vi "main.vi"() -> ()   [LabVIEW 2023]
uses:
  <vilib>/express/express signal manip/GetorSetDDTAttributes/Shared VIs/TimeType.ctl
  5948bca3-3d14-40bf-9fbb-2ba5c3eee3bd.vi
  <vilib>/Analysis/baseanly.llb/Mean (DBL).vi
  faa81322-6883-41b3-8229-1eb533283c0b.vi
  <extravilib>/ChannelInstances/Tag-bool/Read With Abort.vi
  <extravilib>/ChannelInstances/Tag-bool/Write With Abort.vi
  <extravilib>/ChannelInstances/Tag-bool/Instantiate.vi
  <extravilib>/ChannelInstances/Tag-bool/EndpointRead.vi
  <vilib>/express/express signal manip/GetorSetDDTAttributes/Shared VIs/TimeMode Enum to Boolean.vi
  <vilib>/express/express shared/transition.llb/Dynamic To Waveform Array.vi
  <vilib>/express/express signal manip/GetorSetDDTAttributes/Set DDT Attributes/SetT0.vi
  <vilib>/express/express shared/transition.llb/Waveform Array To Dynamic.vi
  <extravilib>/ChannelInstances/Tag-bool/Endpoint.vi
  <vilib>/express/express signal manip/GetorSetDDTAttributes/Set DDT Attributes/Set DDT Properties.xnode
  <extravilib>/ChannelInstances/Tag-bool.lvlib
  <vilib>/ptbypt/NI_PtbyPt.lvlib
  <vilib>/Analysis/NI_AALBase.lvlib
  <vilib>/express/express signal manip/GetorSetDDTAttributes/Shared VIs/GetSetShared.lvlib
panel:
  out "dt":dbl
  in  "?":T1(tab)
  in  "Test Knob":dbl(knob) scale=0.0..10.0
  out "Signal Frequency\n 2":dbl(graph)
  out "Stable RPM measurement?":bool
  in  "Nominal R":dbl
  in  "Nominal Omega":dbl
  in  "Sample rate":dbl=1000.0
  in  "Number of Samples":dbl=5.0
  in  "Voltage Threshold":dbl=0.5
  in  "Number of magnets":dbl=1.0
  out "Omega [RPM]":dbl(knob) scale=0.0..2000.0
  out "Voltage RMS [V]":dbl(knob) scale=0.0..20.0
  out "Power Output [W]":dbl(knob) scale=0.0..20.0
  out "Current RMS [A]":dbl(knob) scale=0.0..20.0
  in  "Button":bool
  out "Signal\nFrequency (Hz)":dbl
  in  "?":bool
  in  "Button 2":bool
  out "Python Error Status":errorcluster
  in  "Filename":path=path "C:/Users/johan/OneDrive - Estudiantes ITCR/TEC/ProyectodeGraduacion/LabEolicaControl/rawdata.txt"
  out "Voltage Sensor":dynamicdata(graph)
  out "Current Sensor":dynamicdata(graph)
  out "Hall sensor\n 2":dynamicdata(graph)
  out "Hall sensor":dynamicdata(graph)
  # "Lab Setup"
  # "Post Processing"
  # "Data Monitoring"
  # "Real Time Analysis variables"
  # "Measurement Point"
  # "File I/O"
  # "About:"
  # "Software Requirements:"
  # "This measuring system was designed for data acquisition of \npower, angular speed, and resistance data for small scale HAWT \nand possibly VAWT. These turbines are being researched and \ndeveloped at LIENE (Laboratorio de Investigación en Energía Eólica) \nat ITCR. \n\nThis module runs a simulation of the measurement signals to test code previous to usage"
  # "Python 3.6+  with the following packages:\n-- NumPy\n-- Plotly"
  # "Programmer:"
  # "This software was designed and programmed by: \n-- Johansell Villalobos Cubillo: \n         Engineering Physics student\n&\n--Mauricio Bolivar Gonzalez"
  # "DAQ Equipment: NI-USB-6000"
  # "The equipment pinout diagram is shown below and the pins are used as follows: \n\nAl 0 -- Hall effect sensor\nAl 1 -- Voltage from zenner diode\nAl 2 -- ACS712 20A current sensor\nAl GND -- common ground"
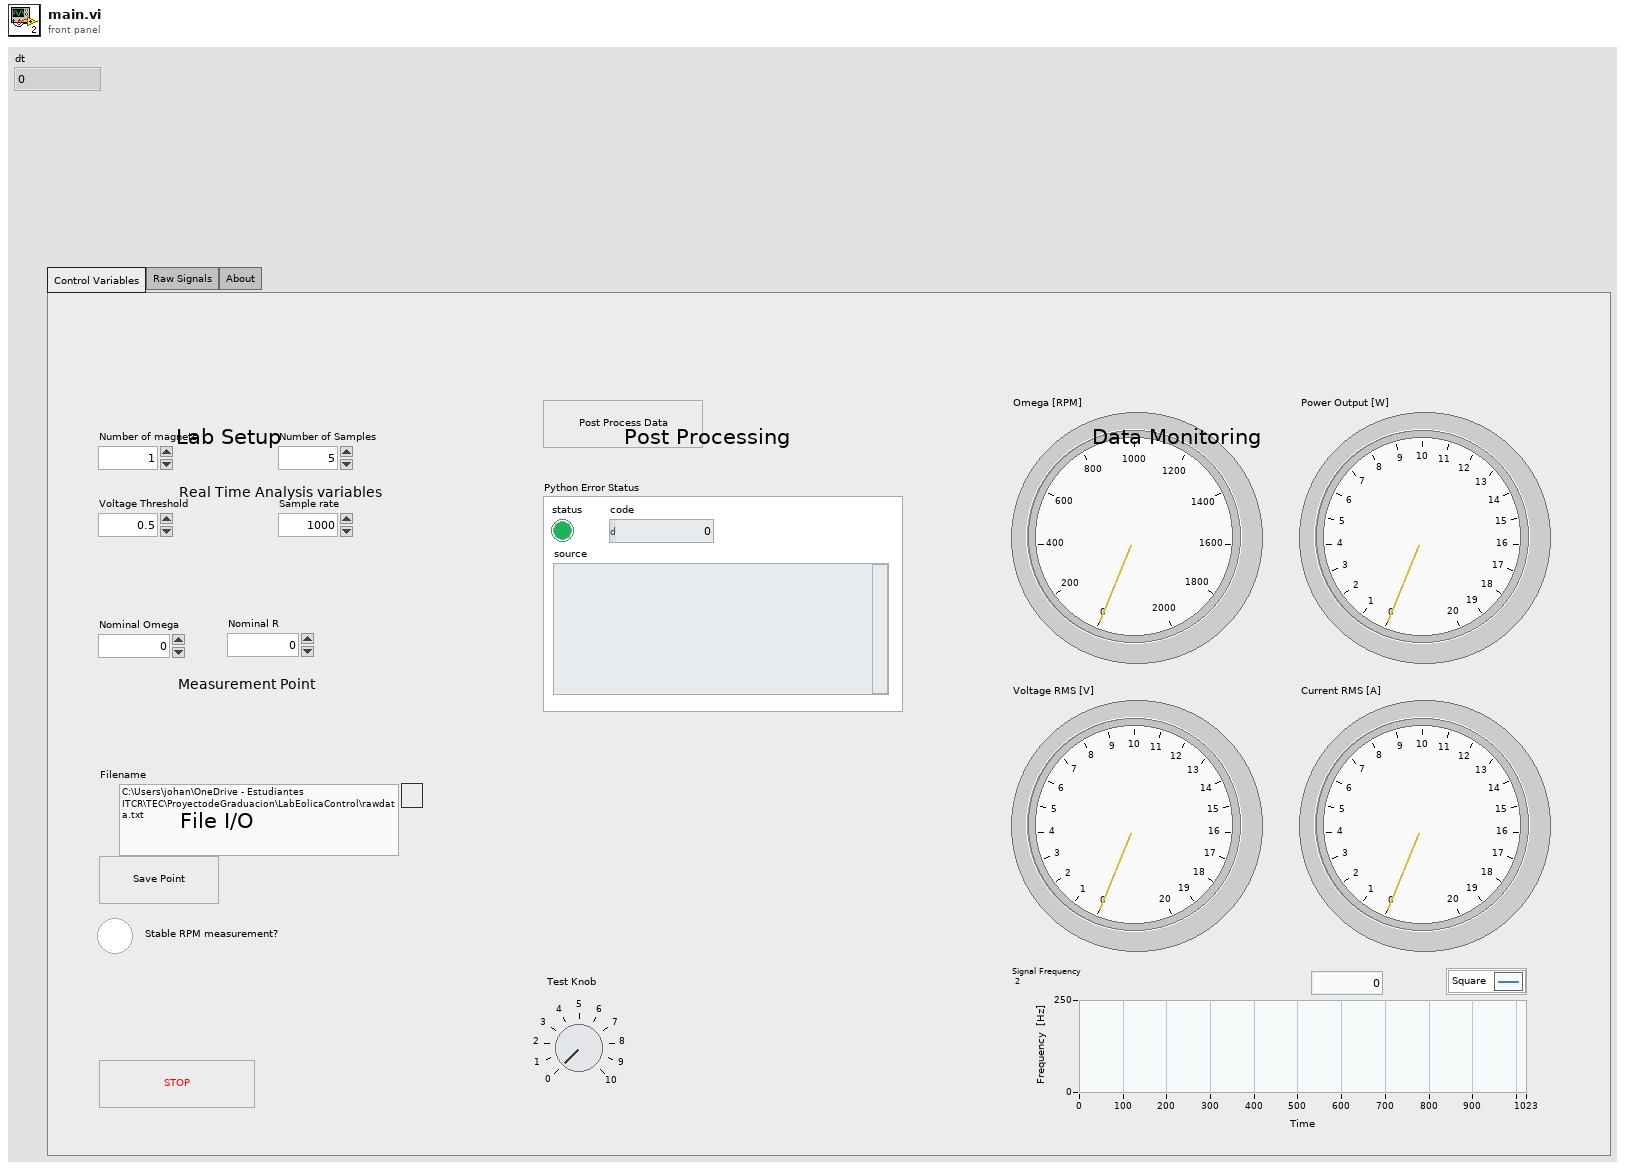
[diagram p1: front panel]
types:
  T1 = enum32{"Control Variables", "Raw Signals", "About"}
  T2 = typedef "Tag-bool.lvlib/))Channel.ctl" = refnum<queue>
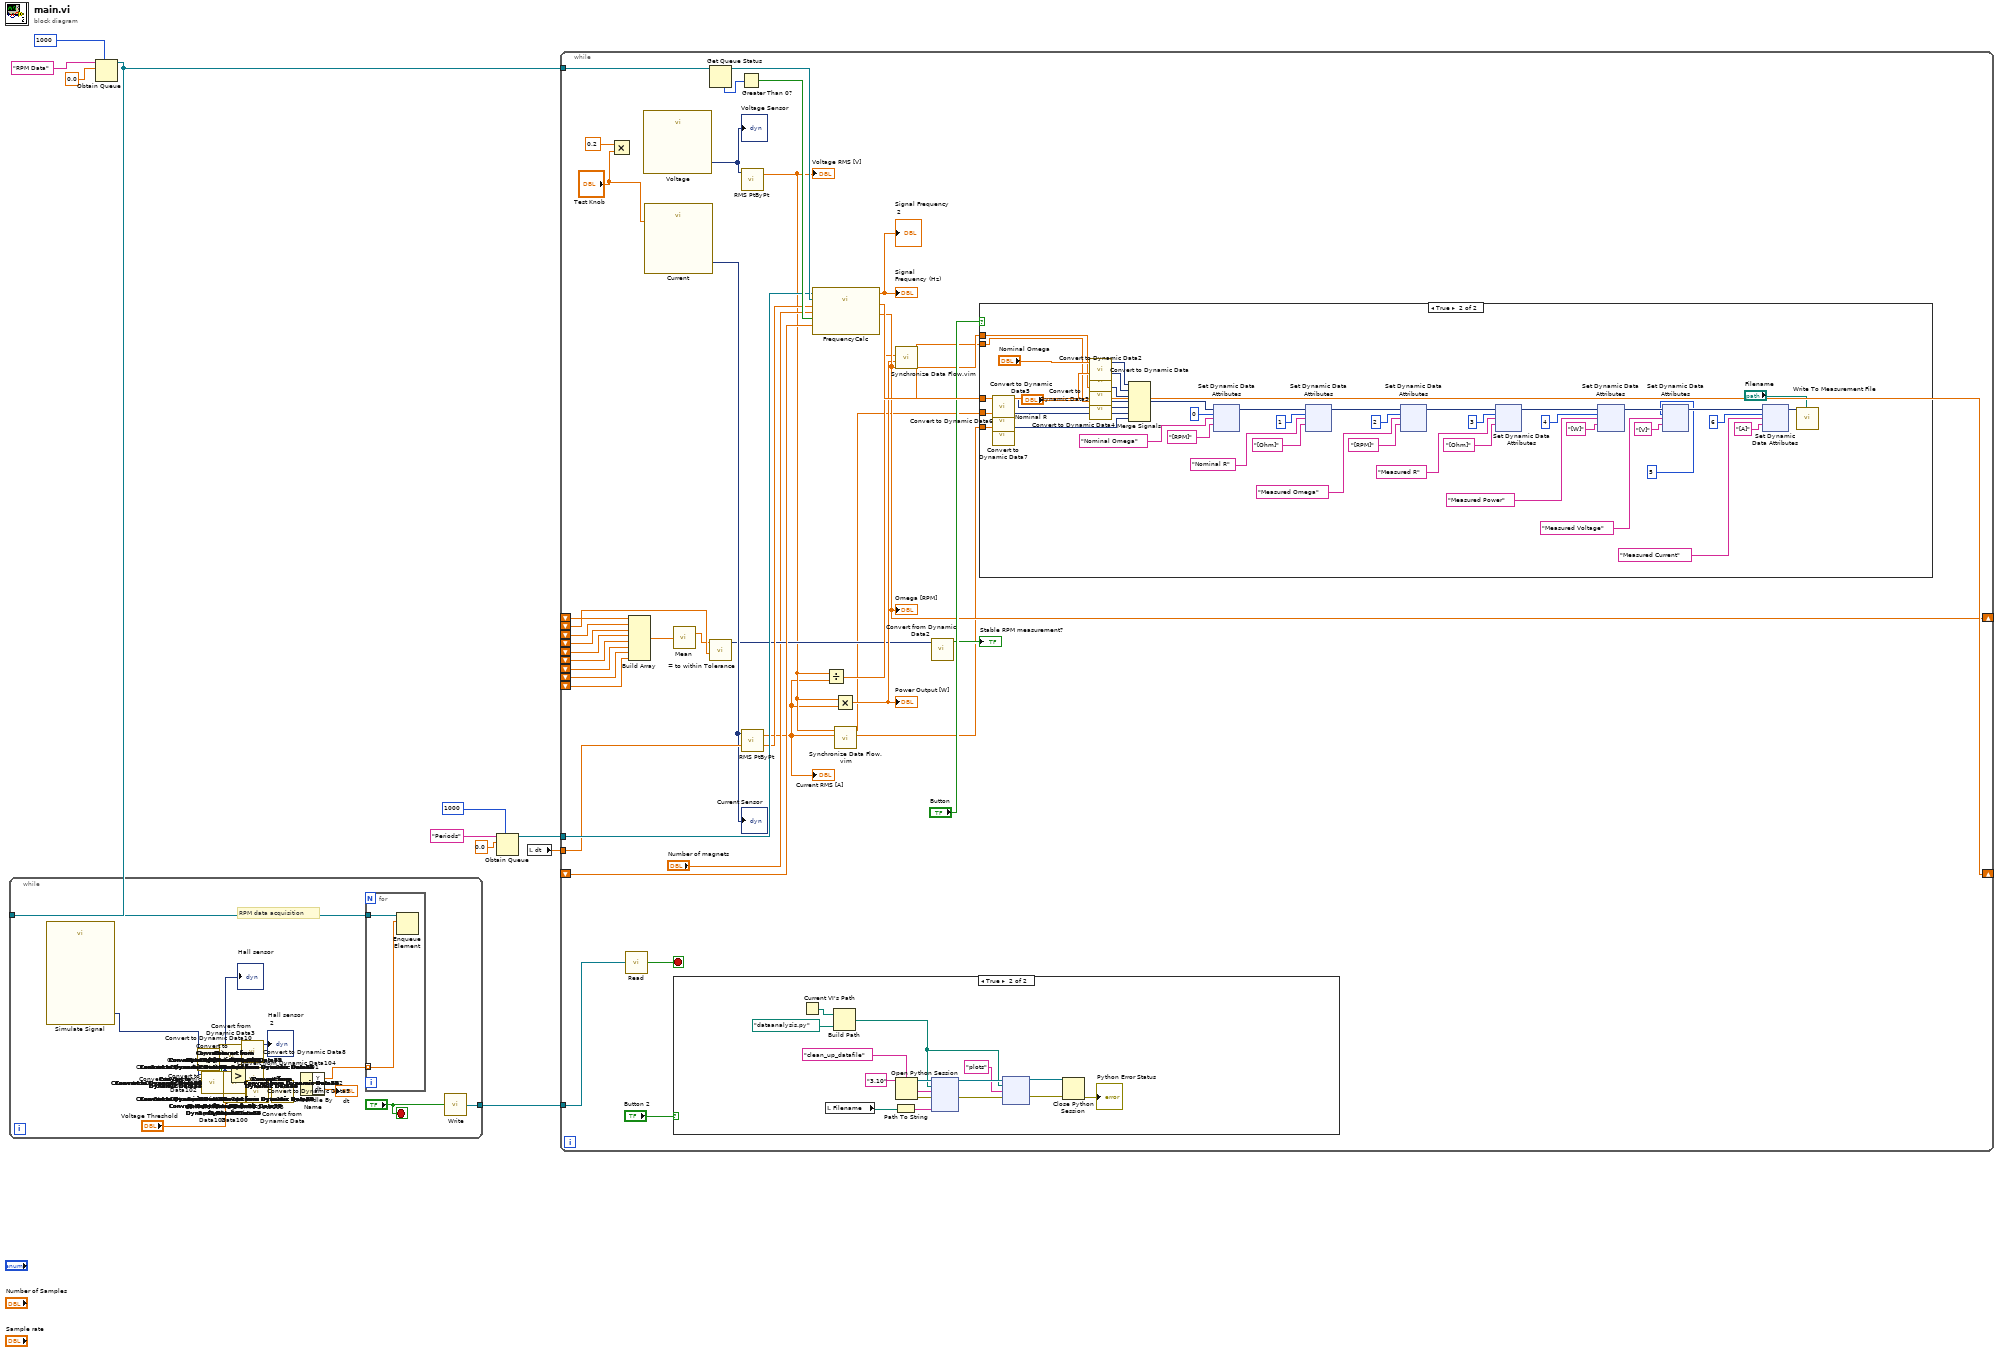
[diagram p0: block diagram]
diagram:
  n1 = Obtain Queue(max queue size (-1, unlimited)=1000 ("max queue size\n(-1, unlimited)"), name (unnamed)="RPM Data" ("name\n(unnamed)"), element data type=0.0 ("data type\n(double)")) -> (queue out=w5:refnum<queue>)  [unwired: 2 in, 2 out]
  n2 = while {
    tunnel: w5 -> [w223]
    tunnel: [w220] -> w7
    stop <- "?" stop-if-true
    # "RPM data acquisition"
    n3 = call "Simulate Signal"() -> ("Square with Uniform Noise"=w215:dynamicdata)  [unwired: 14 in, 1 out]
    "Hall sensor" <- w215
    n4 = Greater?(x=w215, y="Voltage Threshold") -> (0:w221:dynamicdata)
    n5 = call "Convert from Dynamic Data105"("Dynamic Data Type"=w221) -> ("Array"=w11:bool[])  [unwired: 3 in]
    n6 = call "Convert from Dynamic Data104"("Dynamic Data Type"=w221) -> ("Array"=w13:bool[])  [unwired: 3 in]
    n7 = call "Convert to Dynamic Data110"("Array"=w13) -> ("Dynamic Data Type"=w12:dynamicdata)  [unwired: 3 in]
    n8 = call "Convert from Dynamic Data103"("Dynamic Data Type"=w12) -> ("Array"=w15:bool[])  [unwired: 3 in]
    n9 = call "Convert to Dynamic Data109"("Array"=w15) -> ("Dynamic Data Type"=w14:dynamicdata)  [unwired: 3 in]
    n10 = call "Convert from Dynamic Data102"("Dynamic Data Type"=w14) -> ("Array"=w17:bool[])  [unwired: 3 in]
    n11 = call "Convert to Dynamic Data108"("Array"=w17) -> ("Dynamic Data Type"=w16:dynamicdata)  [unwired: 3 in]
    n12 = call "Convert from Dynamic Data101"("Dynamic Data Type"=w16) -> ("Array"=w19:bool[])  [unwired: 3 in]
    n13 = call "Convert to Dynamic Data107"("Array"=w19) -> ("Dynamic Data Type"=w18:dynamicdata)  [unwired: 3 in]
    n14 = call "Convert from Dynamic Data100"("Dynamic Data Type"=w18) -> ("Array"=w21:bool[])  [unwired: 3 in]
    n15 = call "Convert to Dynamic Data106"("Array"=w21) -> ("Dynamic Data Type"=w20:dynamicdata)  [unwired: 3 in]
    n16 = call "Convert from Dynamic Data99"("Dynamic Data Type"=w20) -> ("Array"=w23:bool[])  [unwired: 3 in]
    n17 = call "Convert to Dynamic Data105"("Array"=w23) -> ("Dynamic Data Type"=w22:dynamicdata)  [unwired: 3 in]
    n18 = call "Convert from Dynamic Data98"("Dynamic Data Type"=w22) -> ("Array"=w25:bool[])  [unwired: 3 in]
    n19 = call "Convert to Dynamic Data104"("Array"=w25) -> ("Dynamic Data Type"=w24:dynamicdata)  [unwired: 3 in]
    n20 = call "Convert from Dynamic Data97"("Dynamic Data Type"=w24) -> ("Array"=w27:bool[])  [unwired: 3 in]
    n21 = call "Convert to Dynamic Data103"("Array"=w27) -> ("Dynamic Data Type"=w26:dynamicdata)  [unwired: 3 in]
    n22 = call "Convert from Dynamic Data96"("Dynamic Data Type"=w26) -> ("Array"=w29:bool[])  [unwired: 3 in]
    n23 = call "Convert to Dynamic Data102"("Array"=w29) -> ("Dynamic Data Type"=w28:dynamicdata)  [unwired: 3 in]
    n24 = call "Convert from Dynamic Data95"("Dynamic Data Type"=w28) -> ("Array"=w31:bool[])  [unwired: 3 in]
    n25 = call "Convert to Dynamic Data101"("Array"=w31) -> ("Dynamic Data Type"=w30:dynamicdata)  [unwired: 3 in]
    n26 = call "Convert from Dynamic Data94"("Dynamic Data Type"=w30) -> ("Array"=w33:bool[])  [unwired: 3 in]
    n27 = call "Convert to Dynamic Data100"("Array"=w33) -> ("Dynamic Data Type"=w32:dynamicdata)  [unwired: 3 in]
    n28 = call "Convert from Dynamic Data93"("Dynamic Data Type"=w32) -> ("Array"=w35:bool[])  [unwired: 3 in]
    n29 = call "Convert to Dynamic Data99"("Array"=w35) -> ("Dynamic Data Type"=w34:dynamicdata)  [unwired: 3 in]
    n30 = call "Convert from Dynamic Data92"("Dynamic Data Type"=w34) -> ("Array"=w37:bool[])  [unwired: 3 in]
    n31 = call "Convert to Dynamic Data98"("Array"=w37) -> ("Dynamic Data Type"=w36:dynamicdata)  [unwired: 3 in]
    n32 = call "Convert from Dynamic Data91"("Dynamic Data Type"=w36) -> ("Array"=w39:bool[])  [unwired: 3 in]
    n33 = call "Convert to Dynamic Data97"("Array"=w39) -> ("Dynamic Data Type"=w38:dynamicdata)  [unwired: 3 in]
    n34 = call "Convert from Dynamic Data90"("Dynamic Data Type"=w38) -> ("Array"=w41:bool[])  [unwired: 3 in]
    n35 = call "Convert to Dynamic Data96"("Array"=w41) -> ("Dynamic Data Type"=w40:dynamicdata)  [unwired: 3 in]
    n36 = call "Convert from Dynamic Data89"("Dynamic Data Type"=w40) -> ("Array"=w43:bool[])  [unwired: 3 in]
    n37 = call "Convert to Dynamic Data95"("Array"=w43) -> ("Dynamic Data Type"=w42:dynamicdata)  [unwired: 3 in]
    n38 = call "Convert from Dynamic Data88"("Dynamic Data Type"=w42) -> ("Array"=w45:bool[])  [unwired: 3 in]
    n39 = call "Convert to Dynamic Data94"("Array"=w45) -> ("Dynamic Data Type"=w44:dynamicdata)  [unwired: 3 in]
    n40 = call "Convert from Dynamic Data87"("Dynamic Data Type"=w44) -> ("Array"=w47:bool[])  [unwired: 3 in]
    n41 = call "Convert to Dynamic Data93"("Array"=w47) -> ("Dynamic Data Type"=w46:dynamicdata)  [unwired: 3 in]
    n42 = call "Convert from Dynamic Data86"("Dynamic Data Type"=w46) -> ("Array"=w49:bool[])  [unwired: 3 in]
    n43 = call "Convert to Dynamic Data92"("Array"=w49) -> ("Dynamic Data Type"=w48:dynamicdata)  [unwired: 3 in]
    n44 = call "Convert from Dynamic Data85"("Dynamic Data Type"=w48) -> ("Array"=w51:bool[])  [unwired: 3 in]
    n45 = call "Convert to Dynamic Data91"("Array"=w51) -> ("Dynamic Data Type"=w50:dynamicdata)  [unwired: 3 in]
    n46 = call "Convert from Dynamic Data84"("Dynamic Data Type"=w50) -> ("Array"=w53:bool[])  [unwired: 3 in]
    n47 = call "Convert to Dynamic Data90"("Array"=w53) -> ("Dynamic Data Type"=w52:dynamicdata)  [unwired: 3 in]
    n48 = call "Convert from Dynamic Data83"("Dynamic Data Type"=w52) -> ("Array"=w55:bool[])  [unwired: 3 in]
    n49 = call "Convert to Dynamic Data89"("Array"=w55) -> ("Dynamic Data Type"=w54:dynamicdata)  [unwired: 3 in]
    n50 = call "Convert from Dynamic Data82"("Dynamic Data Type"=w54) -> ("Array"=w57:bool[])  [unwired: 3 in]
    n51 = call "Convert to Dynamic Data88"("Array"=w57) -> ("Dynamic Data Type"=w56:dynamicdata)  [unwired: 3 in]
    n52 = call "Convert from Dynamic Data81"("Dynamic Data Type"=w56) -> ("Array"=w59:bool[])  [unwired: 3 in]
    n53 = call "Convert to Dynamic Data87"("Array"=w59) -> ("Dynamic Data Type"=w58:dynamicdata)  [unwired: 3 in]
    n54 = call "Convert from Dynamic Data80"("Dynamic Data Type"=w58) -> ("Array"=w61:bool[])  [unwired: 3 in]
    n55 = call "Convert to Dynamic Data86"("Array"=w61) -> ("Dynamic Data Type"=w60:dynamicdata)  [unwired: 3 in]
    n56 = call "Convert from Dynamic Data79"("Dynamic Data Type"=w60) -> ("Array"=w63:bool[])  [unwired: 3 in]
    n57 = call "Convert to Dynamic Data85"("Array"=w63) -> ("Dynamic Data Type"=w62:dynamicdata)  [unwired: 3 in]
    n58 = call "Convert from Dynamic Data78"("Dynamic Data Type"=w62) -> ("Array"=w65:bool[])  [unwired: 3 in]
    n59 = call "Convert to Dynamic Data84"("Array"=w65) -> ("Dynamic Data Type"=w64:dynamicdata)  [unwired: 3 in]
    n60 = call "Convert from Dynamic Data77"("Dynamic Data Type"=w64) -> ("Array"=w67:bool[])  [unwired: 3 in]
    n61 = call "Convert to Dynamic Data83"("Array"=w67) -> ("Dynamic Data Type"=w66:dynamicdata)  [unwired: 3 in]
    n62 = call "Convert from Dynamic Data76"("Dynamic Data Type"=w66) -> ("Array"=w69:bool[])  [unwired: 3 in]
    n63 = call "Convert to Dynamic Data82"("Array"=w69) -> ("Dynamic Data Type"=w68:dynamicdata)  [unwired: 3 in]
    n64 = call "Convert from Dynamic Data75"("Dynamic Data Type"=w68) -> ("Array"=w71:bool[])  [unwired: 3 in]
    n65 = call "Convert to Dynamic Data81"("Array"=w71) -> ("Dynamic Data Type"=w70:dynamicdata)  [unwired: 3 in]
    n66 = call "Convert from Dynamic Data74"("Dynamic Data Type"=w70) -> ("Array"=w73:bool[])  [unwired: 3 in]
    n67 = call "Convert to Dynamic Data80"("Array"=w73) -> ("Dynamic Data Type"=w72:dynamicdata)  [unwired: 3 in]
    n68 = call "Convert from Dynamic Data73"("Dynamic Data Type"=w72) -> ("Array"=w75:bool[])  [unwired: 3 in]
    n69 = call "Convert to Dynamic Data79"("Array"=w75) -> ("Dynamic Data Type"=w74:dynamicdata)  [unwired: 3 in]
    n70 = call "Convert from Dynamic Data72"("Dynamic Data Type"=w74) -> ("Array"=w77:bool[])  [unwired: 3 in]
    n71 = call "Convert to Dynamic Data78"("Array"=w77) -> ("Dynamic Data Type"=w76:dynamicdata)  [unwired: 3 in]
    n72 = call "Convert from Dynamic Data71"("Dynamic Data Type"=w76) -> ("Array"=w79:bool[])  [unwired: 3 in]
    n73 = call "Convert to Dynamic Data77"("Array"=w79) -> ("Dynamic Data Type"=w78:dynamicdata)  [unwired: 3 in]
    n74 = call "Convert from Dynamic Data70"("Dynamic Data Type"=w78) -> ("Array"=w81:bool[])  [unwired: 3 in]
    n75 = call "Convert to Dynamic Data76"("Array"=w81) -> ("Dynamic Data Type"=w80:dynamicdata)  [unwired: 3 in]
    n76 = call "Convert from Dynamic Data69"("Dynamic Data Type"=w80) -> ("Array"=w83:bool[])  [unwired: 3 in]
    n77 = call "Convert to Dynamic Data75"("Array"=w83) -> ("Dynamic Data Type"=w82:dynamicdata)  [unwired: 3 in]
    n78 = call "Convert from Dynamic Data68"("Dynamic Data Type"=w82) -> ("Array"=w85:bool[])  [unwired: 3 in]
    n79 = call "Convert to Dynamic Data74"("Array"=w85) -> ("Dynamic Data Type"=w84:dynamicdata)  [unwired: 3 in]
    n80 = call "Convert from Dynamic Data67"("Dynamic Data Type"=w84) -> ("Array"=w87:bool[])  [unwired: 3 in]
    n81 = call "Convert to Dynamic Data73"("Array"=w87) -> ("Dynamic Data Type"=w86:dynamicdata)  [unwired: 3 in]
    n82 = call "Convert from Dynamic Data66"("Dynamic Data Type"=w86) -> ("Array"=w89:bool[])  [unwired: 3 in]
    n83 = call "Convert to Dynamic Data72"("Array"=w89) -> ("Dynamic Data Type"=w88:dynamicdata)  [unwired: 3 in]
    n84 = call "Convert from Dynamic Data65"("Dynamic Data Type"=w88) -> ("Array"=w91:bool[])  [unwired: 3 in]
    n85 = call "Convert to Dynamic Data71"("Array"=w91) -> ("Dynamic Data Type"=w90:dynamicdata)  [unwired: 3 in]
    n86 = call "Convert from Dynamic Data64"("Dynamic Data Type"=w90) -> ("Array"=w93:bool[])  [unwired: 3 in]
    n87 = call "Convert to Dynamic Data70"("Array"=w93) -> ("Dynamic Data Type"=w92:dynamicdata)  [unwired: 3 in]
    n88 = call "Convert from Dynamic Data63"("Dynamic Data Type"=w92) -> ("Array"=w95:bool[])  [unwired: 3 in]
    n89 = call "Convert to Dynamic Data69"("Array"=w95) -> ("Dynamic Data Type"=w94:dynamicdata)  [unwired: 3 in]
    n90 = call "Convert from Dynamic Data62"("Dynamic Data Type"=w94) -> ("Array"=w97:bool[])  [unwired: 3 in]
    n91 = call "Convert to Dynamic Data68"("Array"=w97) -> ("Dynamic Data Type"=w96:dynamicdata)  [unwired: 3 in]
    n92 = call "Convert from Dynamic Data61"("Dynamic Data Type"=w96) -> ("Array"=w99:bool[])  [unwired: 3 in]
    n93 = call "Convert to Dynamic Data67"("Array"=w99) -> ("Dynamic Data Type"=w98:dynamicdata)  [unwired: 3 in]
    n94 = call "Convert from Dynamic Data60"("Dynamic Data Type"=w98) -> ("Array"=w101:bool[])  [unwired: 3 in]
    n95 = call "Convert to Dynamic Data66"("Array"=w101) -> ("Dynamic Data Type"=w100:dynamicdata)  [unwired: 3 in]
    n96 = call "Convert from Dynamic Data59"("Dynamic Data Type"=w100) -> ("Array"=w103:bool[])  [unwired: 3 in]
    n97 = call "Convert to Dynamic Data65"("Array"=w103) -> ("Dynamic Data Type"=w102:dynamicdata)  [unwired: 3 in]
    n98 = call "Convert from Dynamic Data58"("Dynamic Data Type"=w102) -> ("Array"=w105:bool[])  [unwired: 3 in]
    n99 = call "Convert to Dynamic Data64"("Array"=w105) -> ("Dynamic Data Type"=w104:dynamicdata)  [unwired: 3 in]
    n100 = call "Convert from Dynamic Data57"("Dynamic Data Type"=w104) -> ("Array"=w107:bool[])  [unwired: 3 in]
    n101 = call "Convert to Dynamic Data63"("Array"=w107) -> ("Dynamic Data Type"=w106:dynamicdata)  [unwired: 3 in]
    n102 = call "Convert from Dynamic Data56"("Dynamic Data Type"=w106) -> ("Array"=w109:bool[])  [unwired: 3 in]
    n103 = call "Convert to Dynamic Data62"("Array"=w109) -> ("Dynamic Data Type"=w108:dynamicdata)  [unwired: 3 in]
    n104 = call "Convert from Dynamic Data55"("Dynamic Data Type"=w108) -> ("Array"=w111:bool[])  [unwired: 3 in]
    n105 = call "Convert to Dynamic Data61"("Array"=w111) -> ("Dynamic Data Type"=w110:dynamicdata)  [unwired: 3 in]
    n106 = call "Convert from Dynamic Data54"("Dynamic Data Type"=w110) -> ("Array"=w113:bool[])  [unwired: 3 in]
    n107 = call "Convert to Dynamic Data60"("Array"=w113) -> ("Dynamic Data Type"=w112:dynamicdata)  [unwired: 3 in]
    n108 = call "Convert from Dynamic Data53"("Dynamic Data Type"=w112) -> ("Array"=w115:bool[])  [unwired: 3 in]
    n109 = call "Convert to Dynamic Data59"("Array"=w115) -> ("Dynamic Data Type"=w114:dynamicdata)  [unwired: 3 in]
    n110 = call "Convert from Dynamic Data52"("Dynamic Data Type"=w114) -> ("Array"=w117:bool[])  [unwired: 3 in]
    n111 = call "Convert to Dynamic Data58"("Array"=w117) -> ("Dynamic Data Type"=w116:dynamicdata)  [unwired: 3 in]
    n112 = call "Convert from Dynamic Data51"("Dynamic Data Type"=w116) -> ("Array"=w119:bool[])  [unwired: 3 in]
    n113 = call "Convert to Dynamic Data57"("Array"=w119) -> ("Dynamic Data Type"=w118:dynamicdata)  [unwired: 3 in]
    n114 = call "Convert from Dynamic Data50"("Dynamic Data Type"=w118) -> ("Array"=w121:bool[])  [unwired: 3 in]
    n115 = call "Convert to Dynamic Data56"("Array"=w121) -> ("Dynamic Data Type"=w120:dynamicdata)  [unwired: 3 in]
    n116 = call "Convert from Dynamic Data49"("Dynamic Data Type"=w120) -> ("Array"=w123:bool[])  [unwired: 3 in]
    n117 = call "Convert to Dynamic Data55"("Array"=w123) -> ("Dynamic Data Type"=w122:dynamicdata)  [unwired: 3 in]
    n118 = call "Convert from Dynamic Data48"("Dynamic Data Type"=w122) -> ("Array"=w125:bool[])  [unwired: 3 in]
    n119 = call "Convert to Dynamic Data54"("Array"=w125) -> ("Dynamic Data Type"=w124:dynamicdata)  [unwired: 3 in]
    n120 = call "Convert from Dynamic Data47"("Dynamic Data Type"=w124) -> ("Array"=w127:bool[])  [unwired: 3 in]
    n121 = call "Convert to Dynamic Data53"("Array"=w127) -> ("Dynamic Data Type"=w126:dynamicdata)  [unwired: 3 in]
    n122 = call "Convert from Dynamic Data46"("Dynamic Data Type"=w126) -> ("Array"=w129:bool[])  [unwired: 3 in]
    n123 = call "Convert to Dynamic Data52"("Array"=w129) -> ("Dynamic Data Type"=w128:dynamicdata)  [unwired: 3 in]
    n124 = call "Convert from Dynamic Data45"("Dynamic Data Type"=w128) -> ("Array"=w131:bool[])  [unwired: 3 in]
    n125 = call "Convert to Dynamic Data51"("Array"=w131) -> ("Dynamic Data Type"=w130:dynamicdata)  [unwired: 3 in]
    n126 = call "Convert from Dynamic Data44"("Dynamic Data Type"=w130) -> ("Array"=w133:bool[])  [unwired: 3 in]
    n127 = call "Convert to Dynamic Data50"("Array"=w133) -> ("Dynamic Data Type"=w132:dynamicdata)  [unwired: 3 in]
    n128 = call "Convert from Dynamic Data43"("Dynamic Data Type"=w132) -> ("Array"=w135:bool[])  [unwired: 3 in]
    n129 = call "Convert to Dynamic Data49"("Array"=w135) -> ("Dynamic Data Type"=w134:dynamicdata)  [unwired: 3 in]
    n130 = call "Convert from Dynamic Data42"("Dynamic Data Type"=w134) -> ("Array"=w137:bool[])  [unwired: 3 in]
    n131 = call "Convert to Dynamic Data48"("Array"=w137) -> ("Dynamic Data Type"=w136:dynamicdata)  [unwired: 3 in]
    n132 = call "Convert from Dynamic Data41"("Dynamic Data Type"=w136) -> ("Array"=w139:bool[])  [unwired: 3 in]
    n133 = call "Convert to Dynamic Data47"("Array"=w139) -> ("Dynamic Data Type"=w138:dynamicdata)  [unwired: 3 in]
    n134 = call "Convert from Dynamic Data40"("Dynamic Data Type"=w138) -> ("Array"=w141:bool[])  [unwired: 3 in]
    n135 = call "Convert to Dynamic Data46"("Array"=w141) -> ("Dynamic Data Type"=w140:dynamicdata)  [unwired: 3 in]
    n136 = call "Convert from Dynamic Data39"("Dynamic Data Type"=w140) -> ("Array"=w143:bool[])  [unwired: 3 in]
    n137 = call "Convert to Dynamic Data45"("Array"=w143) -> ("Dynamic Data Type"=w142:dynamicdata)  [unwired: 3 in]
    n138 = call "Convert from Dynamic Data38"("Dynamic Data Type"=w142) -> ("Array"=w145:bool[])  [unwired: 3 in]
    n139 = call "Convert to Dynamic Data44"("Array"=w145) -> ("Dynamic Data Type"=w144:dynamicdata)  [unwired: 3 in]
    n140 = call "Convert from Dynamic Data37"("Dynamic Data Type"=w144) -> ("Array"=w147:bool[])  [unwired: 3 in]
    n141 = call "Convert to Dynamic Data43"("Array"=w147) -> ("Dynamic Data Type"=w146:dynamicdata)  [unwired: 3 in]
    n142 = call "Convert from Dynamic Data36"("Dynamic Data Type"=w146) -> ("Array"=w149:bool[])  [unwired: 3 in]
    n143 = call "Convert to Dynamic Data42"("Array"=w149) -> ("Dynamic Data Type"=w148:dynamicdata)  [unwired: 3 in]
    n144 = call "Convert from Dynamic Data35"("Dynamic Data Type"=w148) -> ("Array"=w151:bool[])  [unwired: 3 in]
    n145 = call "Convert to Dynamic Data41"("Array"=w151) -> ("Dynamic Data Type"=w150:dynamicdata)  [unwired: 3 in]
    n146 = call "Convert from Dynamic Data34"("Dynamic Data Type"=w150) -> ("Array"=w153:bool[])  [unwired: 3 in]
    n147 = call "Convert to Dynamic Data40"("Array"=w153) -> ("Dynamic Data Type"=w152:dynamicdata)  [unwired: 3 in]
    n148 = call "Convert from Dynamic Data33"("Dynamic Data Type"=w152) -> ("Array"=w155:bool[])  [unwired: 3 in]
    n149 = call "Convert to Dynamic Data39"("Array"=w155) -> ("Dynamic Data Type"=w154:dynamicdata)  [unwired: 3 in]
    n150 = call "Convert from Dynamic Data32"("Dynamic Data Type"=w154) -> ("Array"=w157:bool[])  [unwired: 3 in]
    n151 = call "Convert to Dynamic Data38"("Array"=w157) -> ("Dynamic Data Type"=w156:dynamicdata)  [unwired: 3 in]
    n152 = call "Convert from Dynamic Data31"("Dynamic Data Type"=w156) -> ("Array"=w159:bool[])  [unwired: 3 in]
    n153 = call "Convert to Dynamic Data37"("Array"=w159) -> ("Dynamic Data Type"=w158:dynamicdata)  [unwired: 3 in]
    n154 = call "Convert from Dynamic Data30"("Dynamic Data Type"=w158) -> ("Array"=w161:bool[])  [unwired: 3 in]
    n155 = call "Convert to Dynamic Data36"("Array"=w161) -> ("Dynamic Data Type"=w160:dynamicdata)  [unwired: 3 in]
    n156 = call "Convert from Dynamic Data29"("Dynamic Data Type"=w160) -> ("Array"=w163:bool[])  [unwired: 3 in]
    n157 = call "Convert to Dynamic Data35"("Array"=w163) -> ("Dynamic Data Type"=w162:dynamicdata)  [unwired: 3 in]
    n158 = call "Convert from Dynamic Data28"("Dynamic Data Type"=w162) -> ("Array"=w165:bool[])  [unwired: 3 in]
    n159 = call "Convert to Dynamic Data34"("Array"=w165) -> ("Dynamic Data Type"=w164:dynamicdata)  [unwired: 3 in]
    n160 = call "Convert from Dynamic Data27"("Dynamic Data Type"=w164) -> ("Array"=w167:bool[])  [unwired: 3 in]
    n161 = call "Convert to Dynamic Data33"("Array"=w167) -> ("Dynamic Data Type"=w166:dynamicdata)  [unwired: 3 in]
    n162 = call "Convert from Dynamic Data26"("Dynamic Data Type"=w166) -> ("Array"=w169:bool[])  [unwired: 3 in]
    n163 = call "Convert to Dynamic Data32"("Array"=w169) -> ("Dynamic Data Type"=w168:dynamicdata)  [unwired: 3 in]
    n164 = call "Convert from Dynamic Data25"("Dynamic Data Type"=w168) -> ("Array"=w171:bool[])  [unwired: 3 in]
    n165 = call "Convert to Dynamic Data31"("Array"=w171) -> ("Dynamic Data Type"=w170:dynamicdata)  [unwired: 3 in]
    n166 = call "Convert from Dynamic Data24"("Dynamic Data Type"=w170) -> ("Array"=w173:bool[])  [unwired: 3 in]
    n167 = call "Convert to Dynamic Data30"("Array"=w173) -> ("Dynamic Data Type"=w172:dynamicdata)  [unwired: 3 in]
    n168 = call "Convert from Dynamic Data23"("Dynamic Data Type"=w172) -> ("Array"=w175:bool[])  [unwired: 3 in]
    n169 = call "Convert to Dynamic Data29"("Array"=w175) -> ("Dynamic Data Type"=w174:dynamicdata)  [unwired: 3 in]
    n170 = call "Convert from Dynamic Data22"("Dynamic Data Type"=w174) -> ("Array"=w177:bool[])  [unwired: 3 in]
    n171 = call "Convert to Dynamic Data28"("Array"=w177) -> ("Dynamic Data Type"=w176:dynamicdata)  [unwired: 3 in]
    n172 = call "Convert from Dynamic Data21"("Dynamic Data Type"=w176) -> ("Array"=w179:bool[])  [unwired: 3 in]
    n173 = call "Convert to Dynamic Data27"("Array"=w179) -> ("Dynamic Data Type"=w178:dynamicdata)  [unwired: 3 in]
    n174 = call "Convert from Dynamic Data20"("Dynamic Data Type"=w178) -> ("Array"=w181:bool[])  [unwired: 3 in]
    n175 = call "Convert to Dynamic Data26"("Array"=w181) -> ("Dynamic Data Type"=w180:dynamicdata)  [unwired: 3 in]
    n176 = call "Convert from Dynamic Data19"("Dynamic Data Type"=w180) -> ("Array"=w183:bool[])  [unwired: 3 in]
    n177 = call "Convert to Dynamic Data25"("Array"=w183) -> ("Dynamic Data Type"=w182:dynamicdata)  [unwired: 3 in]
    n178 = call "Convert from Dynamic Data18"("Dynamic Data Type"=w182) -> ("Array"=w185:bool[])  [unwired: 3 in]
    n179 = call "Convert to Dynamic Data24"("Array"=w185) -> ("Dynamic Data Type"=w184:dynamicdata)  [unwired: 3 in]
    n180 = call "Convert from Dynamic Data17"("Dynamic Data Type"=w184) -> ("Array"=w187:bool[])  [unwired: 3 in]
    n181 = call "Convert to Dynamic Data23"("Array"=w187) -> ("Dynamic Data Type"=w186:dynamicdata)  [unwired: 3 in]
    n182 = call "Convert from Dynamic Data16"("Dynamic Data Type"=w186) -> ("Array"=w189:bool[])  [unwired: 3 in]
    n183 = call "Convert to Dynamic Data22"("Array"=w189) -> ("Dynamic Data Type"=w188:dynamicdata)  [unwired: 3 in]
    n184 = call "Convert from Dynamic Data15"("Dynamic Data Type"=w188) -> ("Array"=w191:bool[])  [unwired: 3 in]
    n185 = call "Convert to Dynamic Data21"("Array"=w191) -> ("Dynamic Data Type"=w190:dynamicdata)  [unwired: 3 in]
    n186 = call "Convert from Dynamic Data14"("Dynamic Data Type"=w190) -> ("Array"=w193:bool[])  [unwired: 3 in]
    n187 = call "Convert to Dynamic Data20"("Array"=w193) -> ("Dynamic Data Type"=w192:dynamicdata)  [unwired: 3 in]
    n188 = call "Convert from Dynamic Data13"("Dynamic Data Type"=w192) -> ("Array"=w195:bool[])  [unwired: 3 in]
    n189 = call "Convert to Dynamic Data19"("Array"=w195) -> ("Dynamic Data Type"=w194:dynamicdata)  [unwired: 3 in]
    n190 = call "Convert from Dynamic Data12"("Dynamic Data Type"=w194) -> ("Array"=w197:bool[])  [unwired: 3 in]
    n191 = call "Convert to Dynamic Data18"("Array"=w197) -> ("Dynamic Data Type"=w196:dynamicdata)  [unwired: 3 in]
    n192 = call "Convert from Dynamic Data11"("Dynamic Data Type"=w196) -> ("Array"=w199:bool[])  [unwired: 3 in]
    n193 = call "Convert to Dynamic Data17"("Array"=w199) -> ("Dynamic Data Type"=w198:dynamicdata)  [unwired: 3 in]
    n194 = call "Convert from Dynamic Data10"("Dynamic Data Type"=w198) -> ("Array"=w201:bool[])  [unwired: 3 in]
    n195 = call "Convert to Dynamic Data16"("Array"=w201) -> ("Dynamic Data Type"=w200:dynamicdata)  [unwired: 3 in]
    n196 = call "Convert from Dynamic Data9"("Dynamic Data Type"=w200) -> ("Array"=w203:bool[])  [unwired: 3 in]
    n197 = call "Convert to Dynamic Data15"("Array"=w203) -> ("Dynamic Data Type"=w202:dynamicdata)  [unwired: 3 in]
    n198 = call "Convert from Dynamic Data8"("Dynamic Data Type"=w202) -> ("Array"=w205:bool[])  [unwired: 3 in]
    n199 = call "Convert to Dynamic Data14"("Array"=w205) -> ("Dynamic Data Type"=w204:dynamicdata)  [unwired: 3 in]
    n200 = call "Convert from Dynamic Data7"("Dynamic Data Type"=w204) -> ("Array"=w207:bool[])  [unwired: 3 in]
    n201 = call "Convert to Dynamic Data13"("Array"=w207) -> ("Dynamic Data Type"=w206:dynamicdata)  [unwired: 3 in]
    n202 = call "Convert from Dynamic Data6"("Dynamic Data Type"=w206) -> ("Array"=w209:bool[])  [unwired: 3 in]
    n203 = call "Convert to Dynamic Data12"("Array"=w209) -> ("Dynamic Data Type"=w208:dynamicdata)  [unwired: 3 in]
    n204 = call "Convert from Dynamic Data5"("Dynamic Data Type"=w208) -> ("Array"=w211:bool[])  [unwired: 3 in]
    n205 = call "Convert to Dynamic Data11"("Array"=w211) -> ("Dynamic Data Type"=w210:dynamicdata)  [unwired: 3 in]
    n206 = call "Convert from Dynamic Data4"("Dynamic Data Type"=w210) -> ("Array"=w213:bool[])  [unwired: 3 in]
    n207 = call "Convert to Dynamic Data10"("Array"=w213) -> ("Dynamic Data Type"=w212:dynamicdata)  [unwired: 3 in]
    n208 = call "Convert from Dynamic Data3"("Dynamic Data Type"=w212) -> ("Array"=w214:bool[])  [unwired: 3 in]
    n209 = call "Convert to Dynamic Data8"("Array"=w214) -> ("Dynamic Data Type"=→"Hall sensor\n 2":dynamicdata)  [unwired: 3 in]
    n210 = call "Convert to Dynamic Data9"("Array"=w11) -> ("Dynamic Data Type"=w216:dynamicdata)  [unwired: 3 in]
    n211 = call "Convert from Dynamic Data"("Dynamic Data Type"=w216) -> ("Waveform"=w225:waveform(dbl))  [unwired: 3 in]
    n212 = Unbundle By Name(w225) -> ("Y"=w224:dbl[], "dt"=→"dt":dbl)
    n213 = for {
      tunnel: w224 -> [w227] mode=indexing
      tunnel: w223 -> [w226]
      n214 = Enqueue Element(queue=w226, element=w227) -> ()  [unwired: 2 in, 3 out]
    }
    n215 = call <extravilib>:"Write.vi"("element"="?") -> ("channel"=w220:T2)  [unwired: 1 out]
  }
  n216 = Obtain Queue(max queue size (-1, unlimited)=1000 ("max queue size\n(-1, unlimited)"), name (unnamed)="Periods" ("name\n(unnamed)"), element data type=0.0 ("data type\n(double)")) -> (queue out=w1:refnum<queue>)  [unwired: 2 in, 2 out]
  n217 = local read "dt"() -> (w6:dbl)
  n218 = while {
    tunnel: w5 -> [w267]
    tunnel: w1 -> [w264]
    shift-right: [w262] -> _
    shift-left: _ -> [w263]
    tunnel: w6 -> [w259]
    tunnel: w7 -> [w260]
    shift-right: [w255] -> _
    shift-left: _ -> [w249]
    shift-left: _ -> [w250]
    shift-left: _ -> [w251]
    shift-left: _ -> [w252]
    shift-left: _ -> [w247]
    shift-left: _ -> [w238]
    shift-left: _ -> [w237]
    shift-left: _ -> [w236]
    shift-left: _ -> [w235]
    stop <- w261 stop-if-true
    n219 = Multiply(x=0.2, y="Test Knob") -> ()  [unwired: 1 out]
    n220 = call <extravilib>:"Read.vi"("channel"=w260) -> ("element"=w261:bool)  [unwired: 1 in, 1 out]
    n221 = Build Array(w252, w251, w250, w249, w238, w237, w236, w235) -> (w248:dbl[])
    n222 = call "Voltage"() -> ("DC with Uniform Noise"=w257:dynamicdata)  [unwired: 14 in, 1 out]
    "Voltage Sensor" <- w257
    n223 = call "Current"("Amplitude"="Test Knob") -> ("Sine"=w258:dynamicdata)  [unwired: 13 in, 1 out]
    "Current Sensor" <- w258
    n224 = call-poly <vilib>:"Mean.vi"("X"=w248) -> ("mean"=w246:dbl)  [unwired: 1 out]
    n225 = case shown="True" "Button 2" {
      frame False {
      }
      frame True {
        n226 = Current VI's Path() -> (path=w276:path)
        n227 = local read "Filename"() -> (w279:path)
        n228 = Build Path(base path=w276, name or relative path=path "dataanalysis.py") -> (appended path=w273:path)
        n229 = Path To String(path=w279) -> (string=w280:string)
        n230 = Open Python Session(python version="3.10" ("Python version")) -> (session out=w281:refnum<k35>, error out=w282:errorcluster)  [unwired: 2 in]
        n231 = node(w281, w273, "clean_up_datafile" ("function name"), w282, w280) -> (w274:refnum<k35>, w271:errorcluster)  [unwired: 3 in, 2 out]
        n232 = node(w274, w273, "plots" ("function name"), w271) -> (w269:refnum<k35>, w270:errorcluster)  [unwired: 2 in, 2 out]
        n233 = Close Python Session(session in=w269, error in=w270) -> (11:→"Python Error Status":errorcluster)
      }
    }
    n234 = Get Queue Status(queue=w267) -> (queue out=w265:refnum<queue>, # elements in queue=w268:i32)  [unwired: 2 in, 6 out]
    n235 = call "= to within Tolerance"("Constant Value to Compare Against"=w247, "Operand 1"=w246) -> ("Result"=w245:dynamicdata)  [unwired: 8 in, 1 out]
    n236 = Greater Than 0?(x=w268) -> (x > 0?=w266:bool)
    n237 = call <vilib>:"RMS PtByPt.vi"("x"=w257) -> ("rms value"=w233:dbl)  [unwired: 3 in, 1 out]
    "Voltage RMS [V]" <- w233
    n238 = call <vilib>:"RMS PtByPt.vi"("x"=w258) -> ("rms value"=w232:dbl)  [unwired: 3 in, 1 out]
    "Current RMS [A]" <- w232
    n239 = call "FrequencyCalc.vi"("Checkbox"=w266, "Number of teeth in gear"="Number of magnets", "Period\n(s) in"=w263, "dt"=w259, "queue in"=w265, "Queue in"=w264) -> ("Omega [RPM]"=w255:dbl, "Period\n(s) out"=w262:dbl, "Signal Frequency (Hz)"=→"Signal\nFrequency (Hz)" →"Signal Frequency\n 2":dbl)  [unwired: 2 in, 1 out]
    "Omega [RPM]" <- w255
    n240 = Divide(x=w233, y=w232) -> (x/y=w254:dbl)
    n241 = Multiply(x=w233, y=w232) -> (x*y=w253:dbl)
    "Power Output [W]" <- w253
    n242 = call "Synchronize Data Flow.vim"("input 2"=w232, "input 1"=w233) -> ("output 2"=w230:dbl, "output 1"=w231:dbl)  [unwired: 2 in, 2 out]
    n243 = call "Synchronize Data Flow.vim"("input 4"=w255, "input 3"=w253, "input 2"=w254) -> ("output 4"=w243:dbl, "output 3"=w241:dbl, "output 2"=w242:dbl)  [unwired: 1 in, 1 out]
    n244 = call "Convert from Dynamic Data2"("Dynamic Data Type"=w245) -> ("Scalar"=→"Stable RPM measurement?":bool)  [unwired: 3 in]
    n245 = case shown="True" "Button" {
      tunnel: w243 -> [_ w322]
      tunnel: w242 -> [_ w323]
      tunnel: w241 -> [_ w318]
      tunnel: w231 -> [_ w296]
      tunnel: w230 -> [_ w295]
      frame False {
      }
      frame True {
        n246 = call "Convert to Dynamic Data5"("Double"=w318) -> ("Dynamic Data Type"=w319:dynamicdata)  [unwired: 3 in]
        n247 = call "Convert to Dynamic Data6"("Double"=w296) -> ("Dynamic Data Type"=w294:dynamicdata)  [unwired: 3 in]
        n248 = call "Convert to Dynamic Data7"("Double"=w295) -> ("Dynamic Data Type"=w293:dynamicdata)  [unwired: 3 in]
        n249 = call "Convert to Dynamic Data"("Double"="Nominal Omega") -> ("Dynamic Data Type"=w325:dynamicdata)  [unwired: 3 in]
        n250 = call "Convert to Dynamic Data2"("Double"="Nominal R") -> ("Dynamic Data Type"=w324:dynamicdata)  [unwired: 3 in]
        n251 = call "Convert to Dynamic Data3"("Double"=w322) -> ("Dynamic Data Type"=w321:dynamicdata)  [unwired: 3 in]
        n252 = call "Convert to Dynamic Data4"("Double"=w323) -> ("Dynamic Data Type"=w320:dynamicdata)  [unwired: 3 in]
        n253 = Merge Signals(w325, w324, w321, w320, w319, w294, w293) -> (w317:dynamicdata)
        n254 = xnode ("Set Dynamic Data Attributes")("Signals In"=w317, "Signal Index"=0, "Signal Name"="Nominal Omega", "Unit"="[RPM]") -> ("Signals Out"=w310:dynamicdata)  [unwired: 3 in, 1 out]
        n255 = xnode ("Set Dynamic Data Attributes")("Signals In"=w310, "Signal Index"=1, "Signal Name"="Nominal R", "Unit"="[Ohm]") -> ("Signals Out"=w306:dynamicdata)  [unwired: 3 in, 1 out]
        n256 = xnode ("Set Dynamic Data Attributes")("Signals In"=w306, "Signal Index"=2, "Signal Name"="Measured Omega", "Unit"="[RPM]") -> ("Signals Out"=w302:dynamicdata)  [unwired: 3 in, 1 out]
        n257 = xnode ("Set Dynamic Data Attributes")("Signals In"=w302, "Signal Index"=3, "Signal Name"="Measured R", "Unit"="[Ohm]") -> ("Signals Out"=w298:dynamicdata)  [unwired: 3 in, 1 out]
        n258 = xnode ("Set Dynamic Data Attributes")("Signals In"=w298, "Signal Index"=4, "Signal Name"="Measured Power", "Unit"="[W]") -> ("Signals Out"=w286:dynamicdata)  [unwired: 3 in, 1 out]
        n259 = xnode ("Set Dynamic Data Attributes")("Signals In"=w286, "Signal Index"=5, "Signal Name"="Measured Voltage", "Unit"="[V]") -> ("Signals Out"=w288:dynamicdata)  [unwired: 3 in, 1 out]
        n260 = xnode ("Set Dynamic Data Attributes")("Signals In"=w288, "Signal Index"=6, "Signal Name"="Measured Current", "Unit"="[A]") -> ("Signals Out"=w285:dynamicdata)  [unwired: 3 in, 1 out]
        n261 = call "Write To Measurement File"("Signals"=w285, "Filename"="Filename") -> ()  [unwired: 15 in, 3 out]
      }
    }
  }
